vi "Execute.vi"(8 "error in":errorcluster, 11 "Set Flows for Blue in":refnum<class "Set Flows for Blue.lvclass">) -> (0 "error out":errorcluster, 1 "Next Step?":bool, 2 "MSG":string, 3 "Set Flows for Blue out":refnum<class "Set Flows for Blue.lvclass">)   [LabVIEW 2013, in "Set Flows for Blue.lvclass"]
uses:
  Set Flows for Blue.lvclass
  Controls/MFC Address.ctl
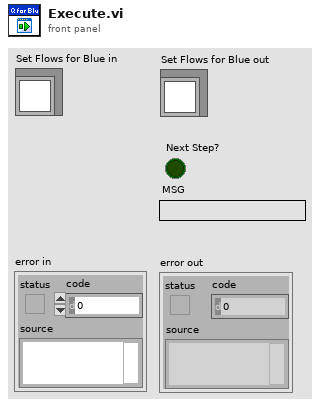
[diagram p1: front panel]
types:
  T1 = typedef "MFC Address.ctl" = enum16{"CRDS Purge", "CRDS Thermodenuded", "CRDS Dry", "CRDS Med RH", "CRDS High RH", "PAS Ch 1", "PAS Ch 2", "PAS Ch3", "PAS Ch 4", "PAS Ch 5", "CLAP", "O3", "Pinlet"}
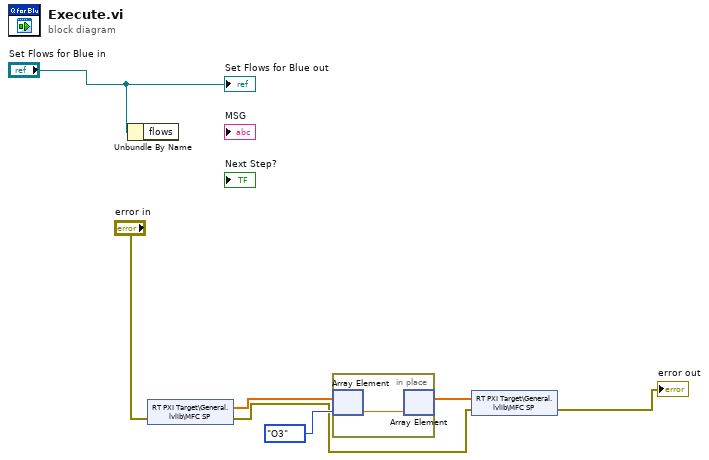
[diagram p0: block diagram]
diagram:
  n1 = Unbundle By Name("Set Flows for Blue in") -> ()  [unwired: 1 out]
  n2 = shared-variable "RT PXI Target\\General.lvlib\\MFC SP"(error in="error in") -> (w7:sgl[], error out=w2:errorcluster)
  n3 = in-place {
    n4 = in-place-array #1(w7, MFC_Address."O3" ("Controllers")) -> (w8:sgl)
    n5 = in-place-array #1(w8) -> (w6:sgl[])  [unwired: 1 out]
  }
  n6 = shared-variable "RT PXI Target\\General.lvlib\\MFC SP"(w6, error in=w2) -> (error out=→"error out":errorcluster)
  "Set Flows for Blue out" <- "Set Flows for Blue in"
